vi "Resistance to Temperature.vi"(8 "error in (no error)":errorcluster, 10 "Resistance In":dbl[](array[numeric]), 11 "2727 in":refnum<class "2727.lvclass">) -> (0 "error out":errorcluster, 2 "Temperature Out":dbl[](array[numeric]), 3 "2727 out":refnum<class "2727.lvclass">)   [LabVIEW 2019, in "2727.lvlib" / "2727.lvclass"]
uses:
  Library/2727.lvclass
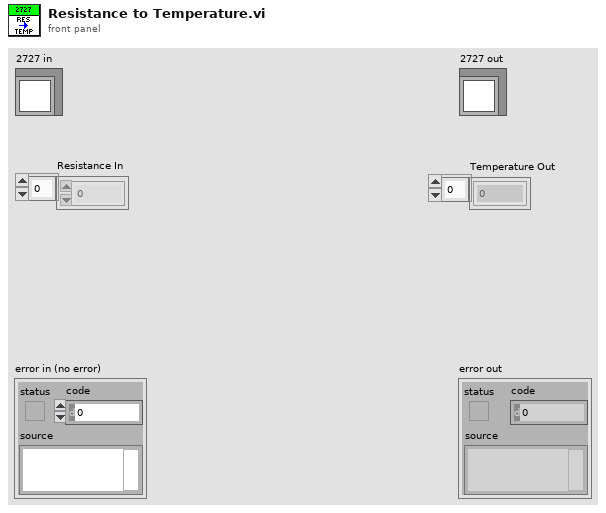
[diagram p1: front panel]
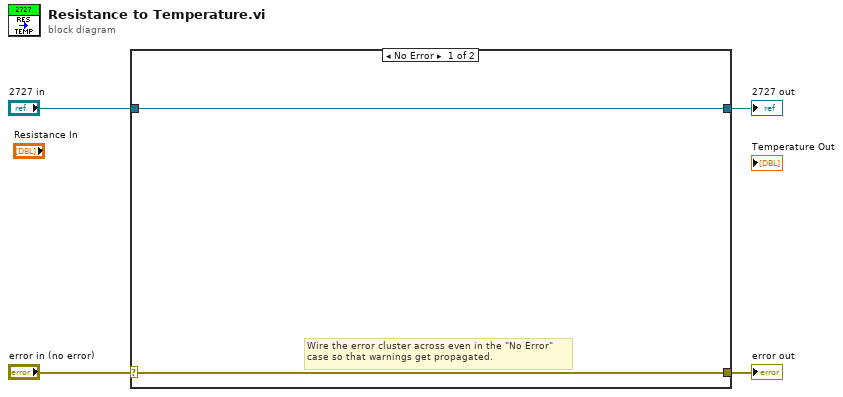
[diagram p0: block diagram]
diagram:
  n1 = case shown="No Error" "error in (no error)" {
    selector: "error in (no error)" -> [w5 w8]
    tunnel: [w5 w8] -> w3
    tunnel: [w6 w7] -> w1
    tunnel: "2727 in" -> [w6 w7]
    frame No Error {
      # "Wire the error cluster across even in the \"No Error\"\ncase so that warnings get propagated."
    }
    frame Error {
    }
  }
  "error out" <- w3
  "2727 out" <- w1
